vi "Autosize Tree Columns.vi"(4 "error in (no error)":errorcluster, 6 "Options":T1={"Whitespace Border"=10, "Resize Table"=FALSE, "Number of Columns"=20, "Default Width"=50}, 7 "Tree Ref":refnum<vi>) -> (0 "error out":errorcluster)   [LabVIEW 2015]
doc: "This VI resizes each column of the Tree specified by Tree Ref based on the widest entry of the column. Additionally, if Resize Tree? is TRUE, the VI will set the Tree width based on the number of populated columns."
panel:
  # "The original code was found in NI Discussion Forum, by ceger\nhttp://forums.ni.com/ni/board/message?board.id=170&message.id=356189\n\nThis version is modified to handle\n1)\tRow's Header column and added default width size for empty Tree.\n2)\tRun from JKI right-click framework\n3)\tChanged control type to Tree."
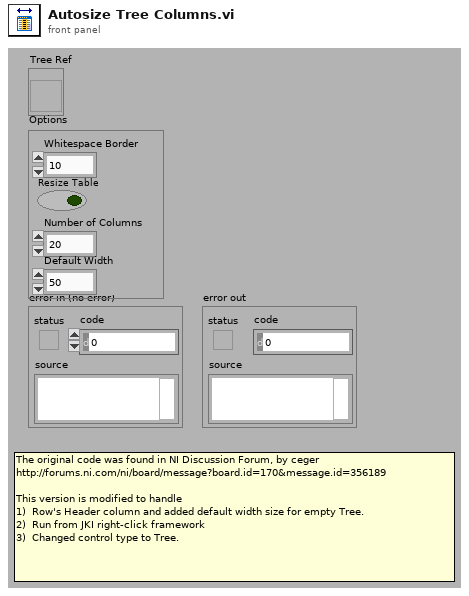
[diagram p1: front panel]
types:
  T1 = cluster{"Whitespace Border":i16, "Resize Table":bool, "Number of Columns":i32, "Default Width":u32}
  T2 = enum16{"User-specified Font", "Application Font", "System Font", "Dialog Font"}
  T3 = cluster{"Font Name:":string, "Size":i16, "Strikeout?":bool, "Italic?":bool, "Underline?":bool, "Outline?":bool, "Shadow?":bool, "Bold?":bool}
  T4 = cluster{"left":i16, "top":i16, "right":i16, "bottom":i16}
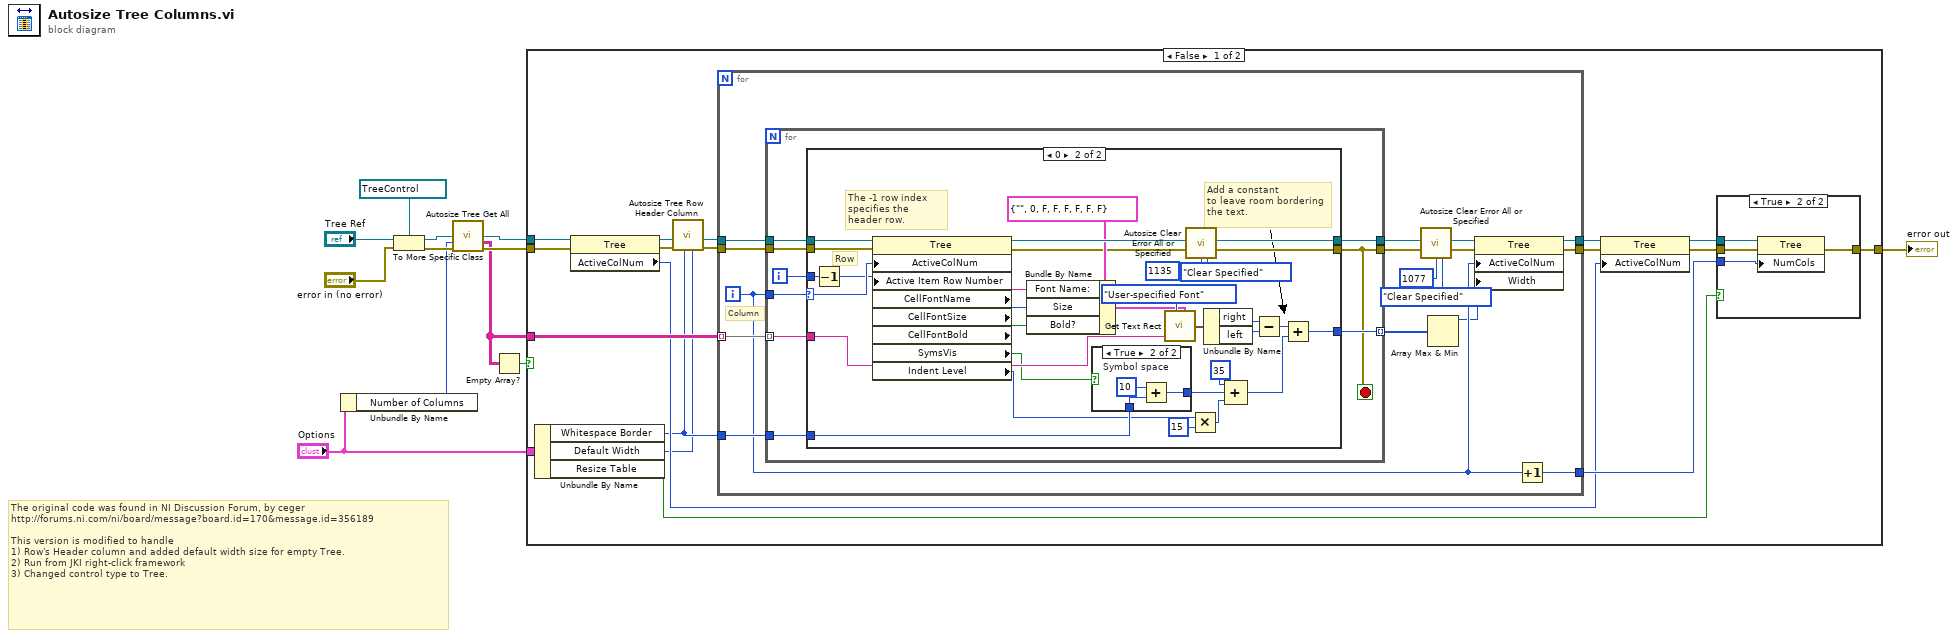
[diagram p0: block diagram]
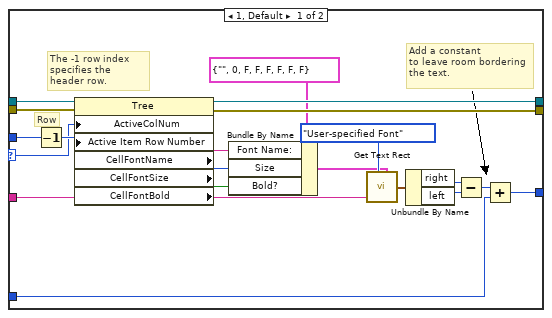
[diagram p3: hidden frame]
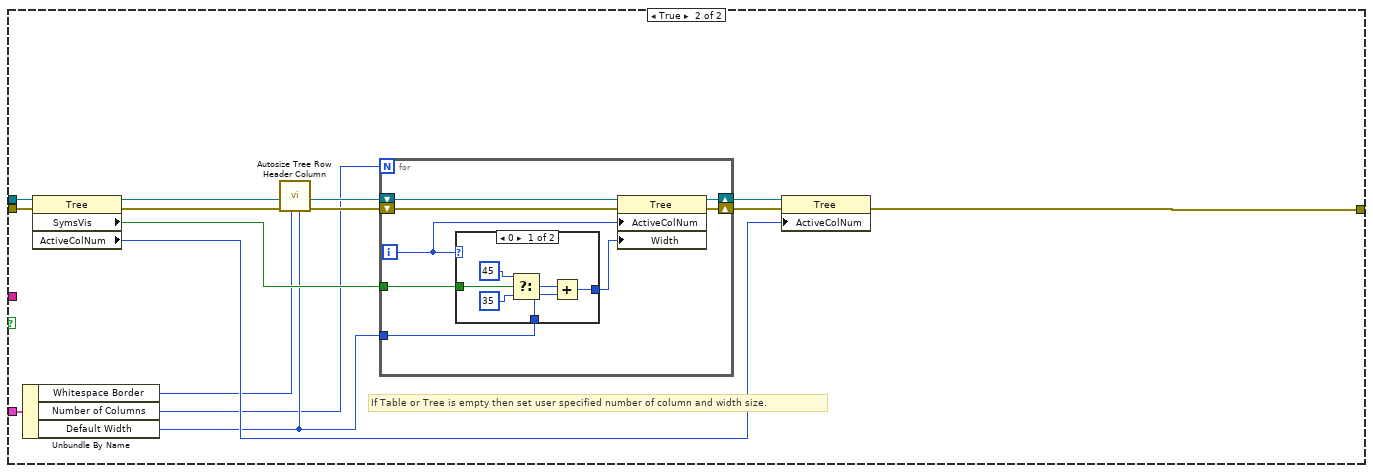
[diagram p5: hidden frame]
diagram:
  # "The original code was found in NI Discussion Forum, by ceger\nhttp://forums.ni.com/ni/board/message?board.id=170&message.id=356189\n\nThis version is modified to handle\n1)\tRow's Header column and added default width size for empty Tree.\n2)\tRun from JKI right-click framework\n3)\tChanged control type to Tree."
  n1 = Unbundle By Name("Options") -> ("Number of Columns"=w1:i32)
  n2 = To More Specific Class(target class=refnum<vi> refnum ("Tree"), reference="Tree Ref", error in="error in (no error)") -> (specific class reference=w4:refnum<vi>, error out=w3:errorcluster)
  n3 = call "Autosize Tree Get All.vi"("Tree Ref"=w4, "Number of Columns"=w1, "error in (no error)"=w3) -> ("Tree Ref out"=w7:refnum<vi>, "Tree Data"=w5:string[][], "error out"=w6:errorcluster)  [unwired: 10 out]
  n4 = Empty Array?(array=w5) -> (empty?=w9:bool)
  n5 = case shown="False" w9 {
    tunnel: w7 -> [w22 w127]
    tunnel: w6 -> [w23 w128]
    tunnel: [w29 w125] -> w12
    tunnel: w5 -> [w28 _]
    tunnel: "Options" -> [w20 w122]
    frame False {
      n6 = Unbundle By Name(w20) -> ("Whitespace Border"=w15:i16, "Default Width"=w13:u32, "Resize Table"=w14:bool)
      n7 = property class="Tree"(reference=w22, error in=w23) -> (reference out=w18:refnum<vi>, error out=w19:errorcluster, "ActiveColNum"=w21:i32)
      n8 = call "Autosize Tree Row Header Column.vi"("Default Width"=w13, "Whitespace Border"=w15, "error in"=w19, "reference in"=w18) -> ("error out"=w16:errorcluster, "reference out"=w17:refnum<vi>)  [unwired: 6 out]
      n9 = for {
        tunnel: w28 -> [w50] mode=indexing
        tunnel: w17 -> [w49]
        tunnel: w16 -> [w47]
        tunnel: [w45] -> w27
        tunnel: [w44] -> w25
        tunnel: [w43] -> w30
        tunnel: w15 -> [w42]
        i -> [w41]
        # "Column"
        n10 = for {
          tunnel: w50 -> [w58] mode=indexing
          tunnel: w49 -> [w59]
          tunnel: w41 -> [w51]
          tunnel: [w55] -> w48 mode=indexing
          tunnel: w47 -> [w57]
          tunnel: [w52] -> w38
          tunnel: [w56] -> w46
          tunnel: w42 -> [w54]
          i -> [w53]
          stop <- w52 stop-if-true
          n11 = case shown="0" w51 {
            selector: w51 -> [w60 w90]
            tunnel: w59 -> [w79 w109]
            tunnel: w58 -> [w78 w108]
            tunnel: w57 -> [w77 w107]
            tunnel: [w76 w106] -> w56
            tunnel: [w75 w105] -> w55
            tunnel: w54 -> [w62 w104]
            tunnel: w53 -> [w74 w85]
            tunnel: [w73 w82] -> w52
            frame 1, Default {
              # "The -1 row index specifies the header row."
              # "Add a constant\nto leave room bordering the text."
              # "Row"
              n12 = Decrement(x=w74) -> (x-1=w61:i32)
              n13 = property class="Tree"(reference=w79, error in=w77, "ActiveColNum"=w60, "Active Item Row Number"=w61) -> (reference out=w76:refnum<vi>, error out=w73:errorcluster, "CellFontName"=w71:string, "CellFontSize"=w63:u32, "CellFontBold"=w70:bool)
              n14 = Bundle By Name(cluster=T3 {"Font Name:"="", "Size"=0, "Strikeout?"=FALSE, "Italic?"=FALSE, "Underline?"=FALSE, "Outline?"=FALSE, "Shadow?"=FALSE, "Bold?"=FALSE} ("[user-specified font]"), "Font Name:"=w71, "Size"=w63, "Bold?"=w70) -> (w68:T3)
              n15 = call <vilib>:"Get Text Rect.vi"("desired font(Application)"=T2."User-specified Font", "text"=w78, "[user-specified font]"=w68) -> ("rect"=w67:T4)  [unwired: 3 in, 3 out]
              n16 = Unbundle By Name(w67) -> ("right"=w66:i16, "left"=w65:i16)
              n17 = Subtract(x=w66, y=w65) -> (x-y=w64:i16)
              n18 = Add(x=w64, y=w62) -> (x+y=w75:i16)
            }
            frame 0 {
              # "The -1 row index specifies the header row."
              # "Add a constant\nto leave room bordering the text."
              # "Row"
              n19 = Decrement(x=w85) -> (x-1=w84:i32)
              n20 = property class="Tree"(reference=w109, error in=w107, "ActiveColNum"=w90, "Active Item Row Number"=w84) -> (reference out=w106:refnum<vi>, error out=w83:errorcluster, "CellFontName"=w102:string, "CellFontSize"=w94:u32, "CellFontBold"=w101:bool, "SymsVis"=w92:bool, "Indent Level"=w91:i32)
              n21 = Bundle By Name(cluster=T3 {"Font Name:"="", "Size"=0, "Strikeout?"=FALSE, "Italic?"=FALSE, "Underline?"=FALSE, "Outline?"=FALSE, "Shadow?"=FALSE, "Bold?"=FALSE} ("[user-specified font]"), "Font Name:"=w102, "Size"=w94, "Bold?"=w101) -> (w99:T3)
              n22 = case shown="True" w92 {
                tunnel: w104 -> [w110 w113]
                tunnel: [w110 w112] -> w88
                frame False {
                }
                frame True {
                  w111 = i16 10  # Symbol space
                  n23 = Add(x=w111, y=w113) -> (x+y=w112:i16)
                }
              }
              n24 = call <vilib>:"Get Text Rect.vi"("desired font(Application)"=T2."User-specified Font", "text"=w108, "[user-specified font]"=w99) -> ("rect"=w98:T4)  [unwired: 3 in, 3 out]
              n25 = call "Autosize Clear Error All or Specified.vi"("Clear Mode (0: Clear All)"=enum16{"Clear All", "Clear Specified"}."Clear Specified", "Code to Clear (0)"=1135, "error in (no error)"=w83) -> ("error out"=w82:errorcluster)  [unwired: 1 in, 11 out]
              n26 = Multiply(x=w91, y=15) -> (x*y=w87:i32)
              n27 = Unbundle By Name(w98) -> ("right"=w97:i16, "left"=w96:i16)
              n28 = Compound Arithmetic op=ADD(i16 35 ("value"), w88, w87) -> (w93:i32)
              n29 = Subtract(x=w97, y=w96) -> (x-y=w95:i16)
              n30 = Add(x=w95, y=w93) -> (x+y=w105:i32)
            }
          }
        }
        n31 = call "Autosize Clear Error All or Specified.vi"("Clear Mode (0: Clear All)"=enum16{"Clear All", "Clear Specified"}."Clear Specified", "Code to Clear (0)"=1077 ("[exception code]"), "error in (no error)"=w38) -> ("error out"=w37:errorcluster)  [unwired: 1 in, 11 out]
        n32 = Array Max & Min(array=w48) -> (max value=w40:i32)  [unwired: 3 out]
        n33 = property class="Tree"(reference=w46, error in=w37, "ActiveColNum"=w41, "Width"=w40) -> (reference out=w44:refnum<vi>, error out=w45:errorcluster)
        n34 = Increment(x=w41) -> (x+1=w43:i32)
      }
      n35 = property class="Tree"(reference=w25, error in=w27, "ActiveColNum"=w21) -> (reference out=w26:refnum<vi>, error out=w24:errorcluster)
      n36 = case shown="True" w14 {
        tunnel: w26 -> [_ w35]
        tunnel: w24 -> [w31 w34]
        tunnel: w30 -> [_ w33]
        tunnel: [w31 w32] -> w29
        frame False {
        }
        frame True {
          n37 = property class="Tree"(reference=w35, error in=w34, "NumCols"=w33) -> (error out=w32:errorcluster)  [unwired: 1 out]
        }
      }
    }
    frame True {
      # "If Table or Tree is empty then set user specified number of column and width size."
      n38 = Unbundle By Name(w122) -> ("Whitespace Border"=w118:i16, "Number of Columns"=w114:i32, "Default Width"=w117:u32)
      n39 = property class="Tree"(reference=w127, error in=w128) -> (reference out=w120:refnum<vi>, error out=w119:errorcluster, "SymsVis"=w126:bool, "ActiveColNum"=w123:i32)
      n40 = call "Autosize Tree Row Header Column.vi"("Default Width"=w117, "Whitespace Border"=w118, "error in"=w119, "reference in"=w120) -> ("error out"=w115:errorcluster, "reference out"=w116:refnum<vi>)  [unwired: 6 out]
      n41 = for {
        N: w114 -> [_]
        tunnel: w126 -> [w129]
        shift-right: [w134] -> w124
        shift-left: w116 -> [w135]
        tunnel: w117 -> [w133]
        shift-right: [w131] -> w121
        shift-left: w115 -> [w132]
        i -> [w130]
        n42 = case shown="0" w130 {
          tunnel: w133 -> [w142 w143]
          tunnel: [w141 w143] -> w136
          tunnel: w129 -> [w140 _]
          frame 0 {
            n43 = Select(t=u32 45 ("x"), s=w140, f=u32 35 ("x")) -> (s? t:f=w138:u32)
            n44 = Add(x=w138, y=w142) -> (x+y=w141:u32)
          }
          frame Default {
          }
        }
        n45 = property class="Tree"(reference=w135, error in=w132, "ActiveColNum"=w130, "Width"=w136) -> (reference out=w134:refnum<vi>, error out=w131:errorcluster)
      }
      n46 = property class="Tree"(reference=w124, error in=w121, "ActiveColNum"=w123) -> (error out=w125:errorcluster)  [unwired: 1 out]
    }
  }
  "error out" <- w12
